vi "DAQmx Create Channel (AI-Temperature-Thermistor-Vex).vi"(0 "task in":refnum<k21>, 1 "maximum value":dbl=100.0 format="%0.2f", 2 "minimum value":dbl format="%0.2f", 3 "resistance configuration":i32(ring)=4 items=["2-Wire"=2, "3-Wire"=3, "4-Wire"=4], 5 "physical channels":tag, 7 "name to assign":string, 9 "units":i32(ring)=10143 items=["Deg C"=10143, "Deg F"=10144, "Kelvins"=10325, "Deg R"=10145, "From Custom Scale"=10065], 10 "voltage excitation value":dbl=2.5 format="%0.5f", 11 "error in":errorcluster, 12 "thermistor characteristics":cluster{"A":dbl, "B":dbl, "C":dbl}={"A"=0.001295361, "B"=0.0002343159, "C"=1.018703e-07} {"C" format="%^0.7e"; "B" format="%^0.7e"; "A" format="%^0.7e"}, 13 "voltage excitation source":i32(ring)=10167 items=["Internal"=10200, "External"=10167, "None"=10230], 14 "r1":dbl=5000.0 format="%0.2f") -> (4 "task out":refnum<k21>, 15 "error out":errorcluster)   [LabVIEW 2013]
doc: "Creates channel(s) that use a thermistor to measure temperature. Use this instance when the thermistor requires voltage excitation."
uses:
  C:/Program Files/National Instruments/LabVIEW 2013/resource/objmgr/daqmx.rc
panel:
  # "input limits"
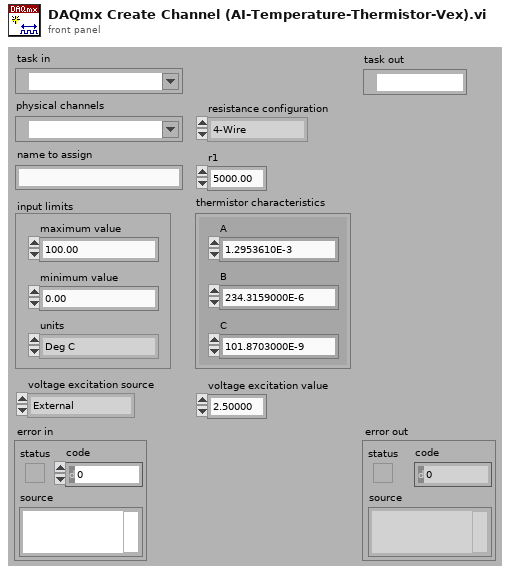
[diagram p1: front panel]
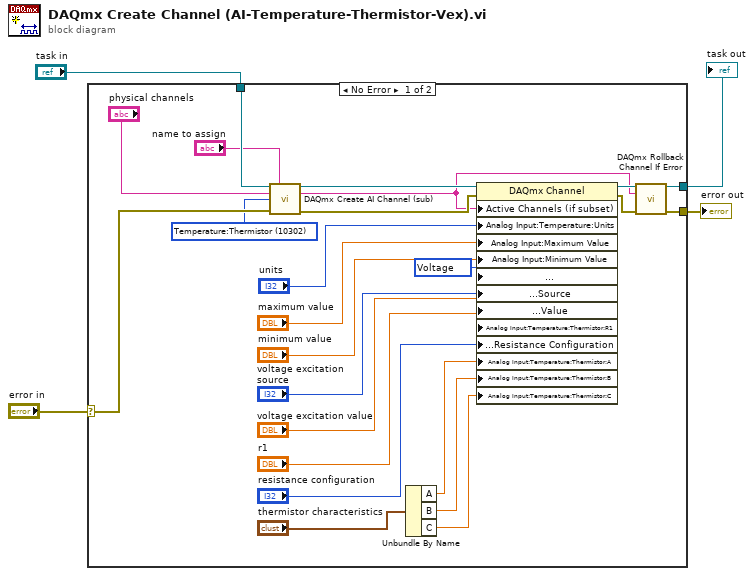
[diagram p0: block diagram]
diagram:
  n1 = case shown="No Error" "error in" {
    selector: "error in" -> [w27 w29]
    tunnel: [w6 w29] -> w4
    tunnel: "task in" -> [w28 w30]
    tunnel: [w7 w30] -> w1
    frame No Error {
      w12 = 10302 items=["Voltage"=10322, "Current"=10134, "More:Voltage:Custom with Excitation"=10323, "More:Current:Custom with Excitation"=10136, "Frequency"=10181, "Period"=10257, "Resistance"=10278, "Temperature:Thermocouple"=10303, "Temperature:Thermistor"=10302, "Temperature:RTD"=10301, "Temperature:Built-in Sensor"=10311, "Strain Gage"=10300] ("measurement type")
      w13 = 10322 items=["Voltage"=10322, "Current"=10134] ("Analog Input:General Properties:Signal Conditioning:Excitation:Advanced:Voltage or Current")
      n2 = call "DAQmx Create AI Channel (sub).vi"("task in"=w28, "virtual channel name"="name to assign", "physical channel name"="physical channels", "measurement type"=w12, "error in"=w27) -> ("task out"=w10:refnum<k21>, "channel names"=w5:string, "error out"=w25:errorcluster)  [unwired: 2 in, 6 out]
      n3 = Unbundle By Name("thermistor characteristics") -> ("A"=w17:dbl, "B"=w16:dbl, "C"=w15:dbl)
      n4 = property class="DAQmx Channel"(reference=w10, error in=w25, "Active Channels (if subset)"=w5, "Analog Input:Temperature:Units"="units", "Analog Input:Maximum Value"="maximum value", "Analog Input:Minimum Value"="minimum value", "Analog Input:General Properties:Signal Conditioning:Excitation:Advanced:Voltage or Current"=w13, "Analog Input:General Properties:Signal Conditioning:Excitation:Source"="voltage excitation source", "Analog Input:General Properties:Signal Conditioning:Excitation:Value"="voltage excitation value", "Analog Input:Temperature:Thermistor:R1"="r1", "Analog Input:General Properties:Signal Conditioning:Resistance Configuration"="resistance configuration", "Analog Input:Temperature:Thermistor:A"=w17, "Analog Input:Temperature:Thermistor:B"=w16, "Analog Input:Temperature:Thermistor:C"=w15) -> (reference out=w9:refnum<k21>, error out=w8:errorcluster)
      n5 = call "DAQmx Rollback Channel If Error.vi"("task in"=w9, "channel names"=w5, "error in"=w8) -> ("task out"=w7:refnum<k21>, "error out"=w6:errorcluster)  [unwired: 11 out]
    }
    frame Error {
    }
  }
  "error out" <- w4
  "task out" <- w1
